vi "BRig_RT__Case_Exp__State_setLaserSettings__v2.vi"(6 "input_FPGA_count2ms":dbl, 7 "input_dataExp":u16[](array[numeric]), 9 "input_dataLC":u16[](array[numeric])) -> (10 "output_LR_nTotal_l1":u32, 12 "output_LR_nTotal_l2":u32, 14 "output_LR_reward_nDelay_l1":u32, 15 "output_LR_wrong_nDelay_l1":u32, 16 "output_LR_reward_nDelay_l2":u32, 17 "output_LR_wrong_nDelay_l2":u32)   [LabVIEW 2014]
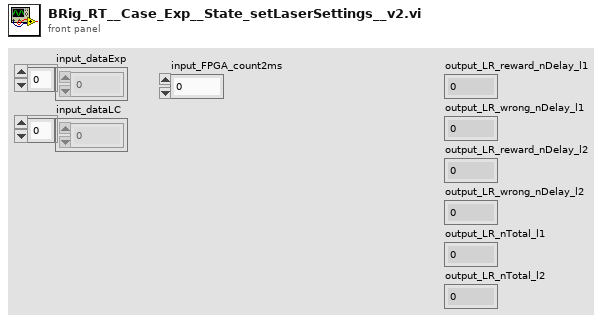
[diagram p1: front panel]
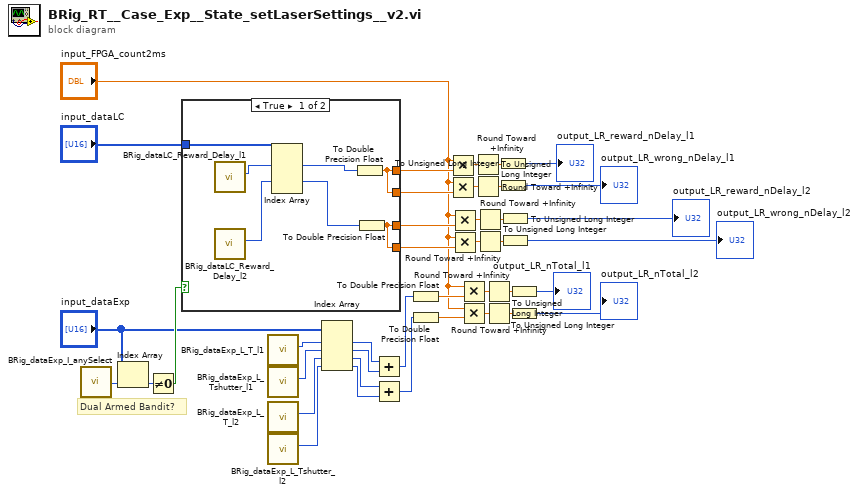
[diagram p0: block diagram]
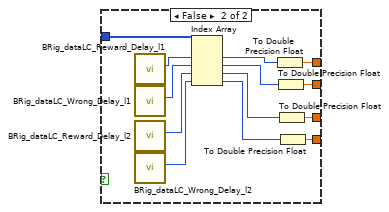
[diagram p2: hidden frame]
diagram:
  # "Dual Armed Bandit?"
  n1 = call "BRig_dataExp_I_anySelect.vi"() -> ("output_I_anySelect"=w1:i32)  [unwired: 11 in]
  n2 = Index Array(array="input_dataExp", index=w1) -> (element=w4:u16)
  n3 = Not Equal To 0?(x=w4) -> (x != 0?=w3:bool)
  n4 = case shown="True" w3 {
    tunnel: [w41 w60] -> w38
    tunnel: [w41 w59] -> w35
    tunnel: [w42 w52] -> w16
    tunnel: [w42 w51] -> w13
    tunnel: "input_dataLC" -> [w43 w48]
    frame True {
      n5 = call "BRig_dataLC_Reward_Delay_l1.vi"() -> ("output_Reward_Delay"=w47:i32)  [unwired: 11 in]
      n6 = call "BRig_dataLC_Reward_Delay_l2.vi"() -> ("output_Reward_Delay_l2"=w46:i32)  [unwired: 11 in]
      n7 = Index Array(array=w43, index #1=w47, index #3=w46) -> (element #1=w45:u16, element #3=w44:u16)  [unwired: 2 in, 2 out]
      n8 = To Double Precision Float(number=w45) -> (double precision float=w41:dbl)
      n9 = To Double Precision Float(number=w44) -> (double precision float=w42:dbl)
    }
    frame False {
      n10 = call "BRig_dataLC_Reward_Delay_l1.vi"() -> ("output_Reward_Delay"=w58:i32)  [unwired: 11 in]
      n11 = call "BRig_dataLC_Wrong_Delay_l1.vi"() -> ("output_Wrong_Delay"=w55:i32)  [unwired: 11 in]
      n12 = call "BRig_dataLC_Reward_Delay_l2.vi"() -> ("output_Reward_Delay_l2"=w56:i32)  [unwired: 11 in]
      n13 = call "BRig_dataLC_Wrong_Delay_l2.vi"() -> ("output_Wrong_Delay_l2"=w57:i32)  [unwired: 11 in]
      n14 = Index Array(array=w48, index #1=w58, index #2=w55, index #3=w56, index #4=w57) -> (element #1=w54:u16, element #2=w53:u16, element #3=w50:u16, element #4=w49:u16)
      n15 = To Double Precision Float(number=w54) -> (double precision float=w60:dbl)
      n16 = To Double Precision Float(number=w53) -> (double precision float=w59:dbl)
      n17 = To Double Precision Float(number=w50) -> (double precision float=w52:dbl)
      n18 = To Double Precision Float(number=w49) -> (double precision float=w51:dbl)
    }
  }
  n19 = call "BRig_dataExp_L_T_l1.vi"() -> ("output_L_T_l1"=w34:i32)  [unwired: 11 in]
  n20 = call "BRig_dataExp_L_Tshutter_l1.vi"() -> ("output_L_Tshutter_l1"=w33:i32)  [unwired: 11 in]
  n21 = call "BRig_dataExp_L_T_l2.vi"() -> ("output_L_T_l2"=w32:i32)  [unwired: 11 in]
  n22 = call "BRig_dataExp_L_Tshutter_l2.vi"() -> ("output_L_Tshutter_l2"=w31:i32)  [unwired: 11 in]
  n23 = Index Array(array="input_dataExp", index #1=w34, index #2=w33, index #3=w32, index #4=w31) -> (element #1=w30:u16, element #2=w29:u16, element #3=w28:u16, element #4=w27:u16)
  n24 = Add(x=w30, y=w29) -> (x+y=w20:u16)
  n25 = Add(x=w28, y=w27) -> (x+y=w19:u16)
  n26 = To Double Precision Float(number=w20) -> (double precision float=w22:dbl)
  n27 = To Double Precision Float(number=w19) -> (double precision float=w21:dbl)
  n28 = Multiply(x="input_FPGA_count2ms", y=w38) -> (x*y=w39:dbl)
  n29 = Multiply(x="input_FPGA_count2ms", y=w35) -> (x*y=w36:dbl)
  n30 = Multiply(x="input_FPGA_count2ms", y=w16) -> (x*y=w17:dbl)
  n31 = Multiply(x="input_FPGA_count2ms", y=w13) -> (x*y=w14:dbl)
  n32 = Multiply(x="input_FPGA_count2ms", y=w22) -> (x*y=w24:dbl)
  n33 = Multiply(x="input_FPGA_count2ms", y=w21) -> (x*y=w26:dbl)
  n34 = Round Toward +Infinity(x=w39) -> (ceil(x): smallest int >= x=w40:dbl)
  n35 = Round Toward +Infinity(x=w36) -> (ceil(x): smallest int >= x=w37:dbl)
  n36 = Round Toward +Infinity(x=w17) -> (ceil(x): smallest int >= x=w18:dbl)
  n37 = Round Toward +Infinity(x=w14) -> (ceil(x): smallest int >= x=w15:dbl)
  n38 = Round Toward +Infinity(x=w24) -> (ceil(x): smallest int >= x=w23:dbl)
  n39 = Round Toward +Infinity(x=w26) -> (ceil(x): smallest int >= x=w25:dbl)
  n40 = To Unsigned Long Integer(number=w40) -> (unsigned 32bit integer=→"output_LR_reward_nDelay_l1":u32)
  n41 = To Unsigned Long Integer(number=w37) -> (unsigned 32bit integer=→"output_LR_wrong_nDelay_l1":u32)
  n42 = To Unsigned Long Integer(number=w18) -> (unsigned 32bit integer=→"output_LR_reward_nDelay_l2":u32)
  n43 = To Unsigned Long Integer(number=w15) -> (unsigned 32bit integer=→"output_LR_wrong_nDelay_l2":u32)
  n44 = To Unsigned Long Integer(number=w23) -> (unsigned 32bit integer=→"output_LR_nTotal_l1":u32)
  n45 = To Unsigned Long Integer(number=w25) -> (unsigned 32bit integer=→"output_LR_nTotal_l2":u32)
